vi "Turret_Globals.vi"() -> ()   [LabVIEW 2019]
uses:
  Turret_Cluster.ctl
  Turret_States.ctl
  Utility_VIs/Basic_Motor_Modes.ctl
panel:
  in  "Turret_Spin_Output":dbl
  in  "Motor_Mode":T1
  out "Turret_Locked":bool
  in  "Turret_CANcoder":string="Turret_CANcoder"
  in  "Turret_Spin":string="Turret_Spin"
  in  "Turret_Execute_Notifier":refnum<notifier>
  in  "Turret_Set_Notifier":refnum<notifier>
  in  "Turret_Execute_Ref":string="Turret_Execute_Ref"
  in  "Turret_Set_Ref":string="Turret_Set_Ref"
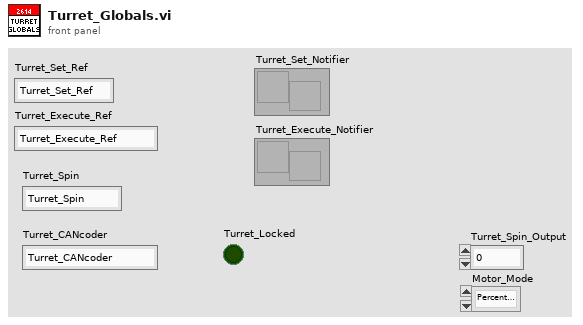
[diagram p1: front panel]
types:
  T1 = typedef "Basic_Motor_Modes.ctl" = enum16{"Percent_Voltage", "Speed_Control", "Position_Control", "Current"}
diagram:
